vi "ExtractMethods.vi"(0 "Method":T2, 1 "Input Array":string[][](array[string]), 5 "Property":T2, 7 "URL":T2, 9 "Data Type":T2, 11 "Error In":errorcluster, 12 "Display?":T2) -> (4 "Complete filtered array":string[][][](array[string]), 6 "Meth/Prop/URL/Type/Disp?":T1(array[cluster]), 15 "Error Out":errorcluster)   [LabVIEW 2014]
uses:
  Controls/ColumnHeaders1.ctl
  Controls/MethodType.ctl
  Tables/scan_array.llb/Scan Array (I32).vi
panel:
  out "Display":string[](array[string])
  out "Output Property":string[](array[string])
  out "Output Types":string[](array[string])
  out "Output URLS":string[](array[string])
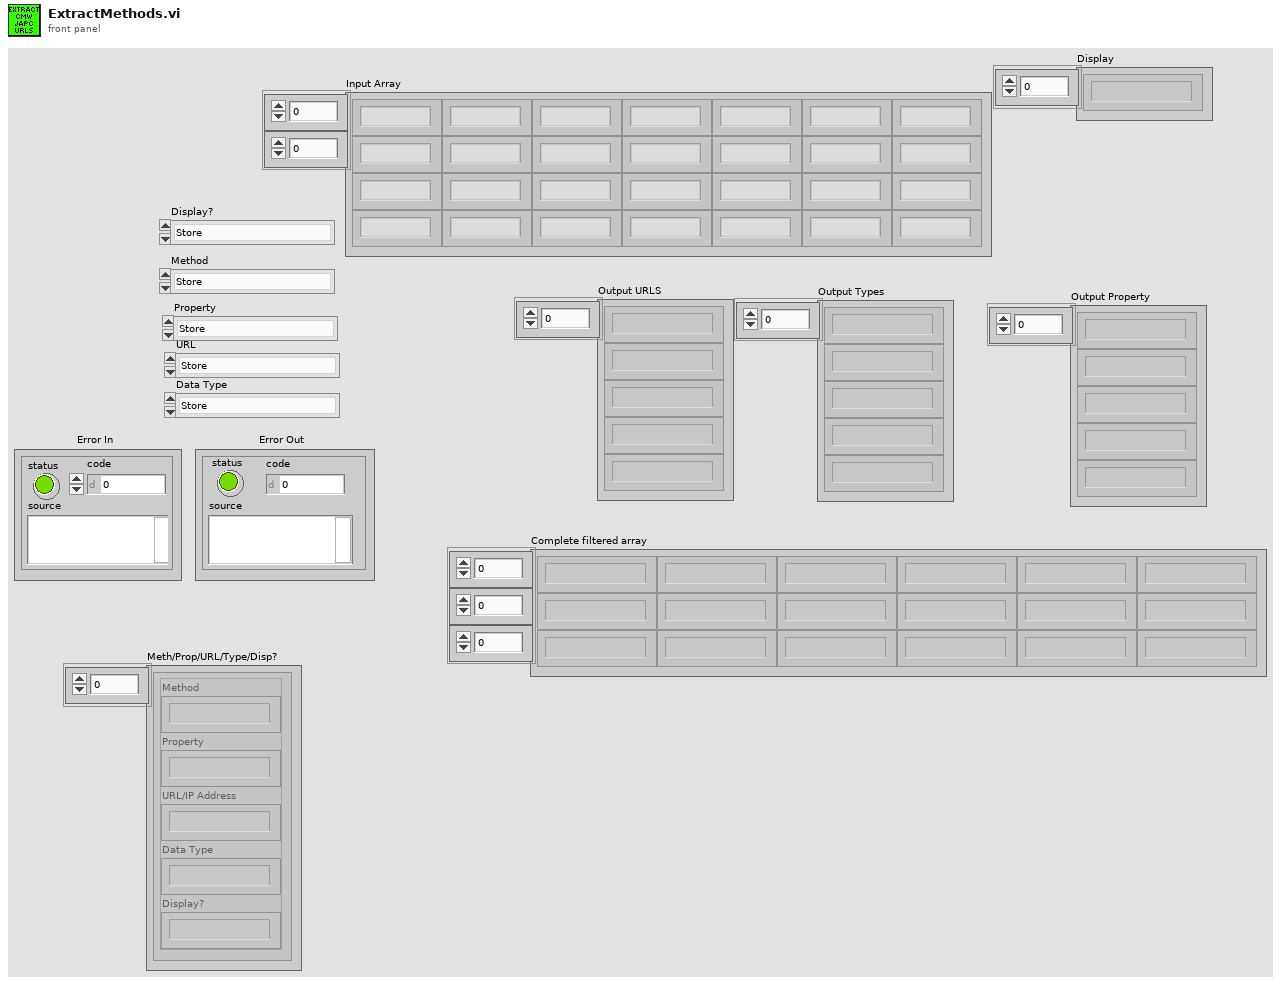
[diagram p1: front panel]
types:
  T1 = cluster{"Method":string, "Property":string, "URL/IP Address":string, "Data Type":string, "Display?":string}[]
  T2 = typedef "ColumnHeaders1.ctl" = enum16{"Store", "Display", "Method", "Property", "Unit", "URL", "IP Address", "Slot", "Address", "Data Type"}
  T3 = typedef "MethodType.ctl" = enum16{"CMW", "JAPC", "PLC"}
  T4 = cluster{"String":string, "String":string, "String":string, "String":string, "String":string}[]
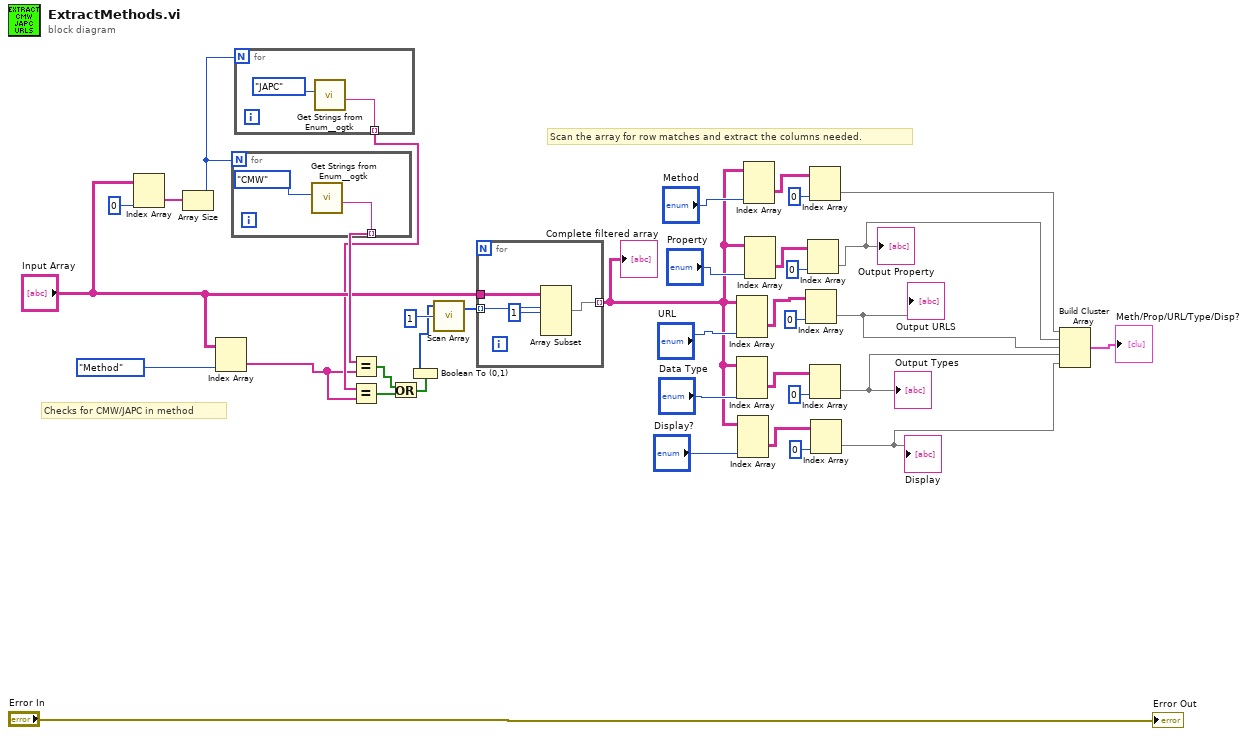
[diagram p0: block diagram]
diagram:
  # "Checks for CMW/JAPC in method"
  # "Scan the array for row matches and extract the columns needed."
  n1 = Index Array(array="Input Array", index (col)=0 ("disabled index (col)")) -> (element=w30:string[])  [unwired: 1 in]
  n2 = Array Size(array=w30) -> (size(s)=w16:i32)
  n3 = Index Array(array="Input Array", index (col)=ColumnHeaders1."Method" ("ColumnHeaders")) -> (element=w14:string[])  [unwired: 1 in]
  n4 = for {
    N: w16 -> [_]
    tunnel: [w38] -> w31 mode=indexing
    n5 = call <userlib>:"Get Strings from Enum__ogtk.vi"("Enum"=MethodType."CMW") -> ("String Value"=w38:string)  [unwired: 7 in, 3 out]
  }
  n6 = for {
    N: w16 -> [_]
    tunnel: [w40] -> w15 mode=indexing
    n7 = call <userlib>:"Get Strings from Enum__ogtk.vi"("Enum"=MethodType."JAPC" ("Enum 2")) -> ("String Value"=w40:string)  [unwired: 7 in, 3 out]
  }
  n8 = Equal?(x=w31, y=w14) -> (x = y?=w12:bool[])
  n9 = Equal?(x=w15, y=w14) -> (x = y?=w13:bool[])
  n10 = Or(x=w12, y=w13) -> (x .or. y?=w11:bool[])
  n11 = Boolean To (0,1)(Boolean=w11) -> (0, 1=w35:i16[])
  n12 = call-poly "Scan Array.vi"("search element"=1, "Input array"=w35) -> ("Matched Indices"=w37:i32[])  [unwired: 3 in]
  n13 = for {
    tunnel: w37 -> [w45] mode=indexing
    tunnel: [w43] -> w3 mode=indexing
    tunnel: "Input Array" -> [w42]
    n14 = Array Subset(array=w42, index (row)=w45, length (row)=1 ("length")) -> (w43:string[][])  [unwired: 2 in]
  }
  "Complete filtered array" <- w3
  n15 = Index Array(array=w3, index (dim 2)="URL") -> (element=w32:string[][])  [unwired: 2 in]
  n16 = Index Array(array=w3, index (dim 2)="Data Type") -> (element=w26:string[][])  [unwired: 2 in]
  n17 = Index Array(array=w3, index (dim 2)="Display?") -> (element=w6:string[][])  [unwired: 2 in]
  n18 = Index Array(array=w3, index (dim 2)="Method") -> (element=w9:string[][])  [unwired: 2 in]
  n19 = Index Array(array=w3, index (dim 2)="Property") -> (element=w21:string[][])  [unwired: 2 in]
  n20 = Index Array(array=w32, index (col)=0) -> (element=w18:string[])  [unwired: 1 in]
  "Output URLS" <- w18
  n21 = Index Array(array=w21, index (col)=0 ("disabled index (col)")) -> (element=w19:string[])  [unwired: 1 in]
  "Output Property" <- w19
  n22 = Index Array(array=w9, index (col)=0) -> (element=w7:string[])  [unwired: 1 in]
  n23 = Index Array(array=w26, index (col)=0) -> (element=w17:string[])  [unwired: 1 in]
  "Output Types" <- w17
  n24 = Index Array(array=w6, index (col)=0) -> (element=w2:string[])  [unwired: 1 in]
  "Display" <- w2
  n25 = Build Cluster Array(w7, w19, w18, w17, w2) -> (→"Meth/Prop/URL/Type/Disp?":T4)
  "Error Out" <- "Error In"
